vi "AFG3352X.set burst mode.vi"(0 "i ref in":refnum<vi>, 1 "Channel (1: 1)":i32(ring)=1 items=["1"=1, "2"=2], 3 "ms timeout (10000)":i32=10000, 4 "Burst Mode \n(0: Triggered)":i32(ring)=1 items=["Triggered", "Gated"], 5 "error in (no error)":errorcluster) -> (14 "i ref out":refnum<vi>, 17 "timed out":bool, 19 "error out":errorcluster)   [LabVIEW 2014, in "AFG3352X.lvlib"]
doc: "Sets the frequency at my device."
uses:
  AFG3352X.lvlib
  CSlibraries/UtilityLib/UtilityLib.valueStatus.ctl
  CSCore/CSApplicationBaseClasses/AFGBase/AFGBase.directionType.ctl
  CSCore/CSApplicationBaseClasses/DeviceBase/DeviceBase.lvlib
  CSinstr.lib/Agilent 3352X Series/Agilent 3352X Series.lvlib
  CSlibraries/UtilityLib/UtilityLib.lvlib
  CSCore/CSApplicationBaseClasses/AFGBase/AFGBase.lvlib
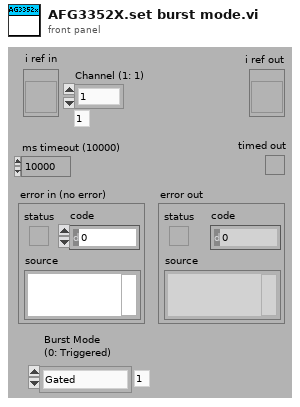
[diagram p1: front panel]
types:
  T1 = typedef "AFGBase.lvlib/AFGBase.directionType.ctl" = enum16{"unknown", "update actual value", "update nominal value", "update both"}
  T2 = typedef "UtilityLib.lvlib/UtilityLib.valueStatus.ctl" = enum16{"no info available", "stand by/off", "on", "warning", "alarm/malfunction", "not implemented", "user action required", "important information", "system default", "control default", "indicator default", "button default"}
  T3 = typedef "AFG3352X.lvlib/AFG3352X.i attribute.ctl" = cluster{"Act2ndValues":cluster{"frequency":dbl, "amplitude":dbl, "phase":dbl, "DCOffset":dbl, "waveformType":T4, "enableOutput":bool, "trigger":i16[], "serviceIDs":cluster{"frequencyID":i32, "amplitudeID":i32, "phaseID":i32, "DCOffsetID":i32, "waveformTypeID":i32, "enableOutputID":i32, "triggerID":i32}, "waveform":cluster{"data":waveform(dbl), "gain":dbl, "offset":dbl, "repetitionRate":dbl, "sampleRate":dbl}}, "Nom2ndValues":cluster{"frequency":dbl, "amplitude":dbl, "phase":dbl, "DCOffset":dbl, "waveformType":T4, "enableOutput":bool, "trigger":i16[], "serviceIDs":cluster{"frequencyID":i32, "amplitudeID":i32, "phaseID":i32, "DCOffsetID":i32, "waveformTypeID":i32, "enableOutputID":i32, "triggerID":i32}, "waveform":cluster{"data":waveform(dbl), "gain":dbl, "offset":dbl, "repetitionRate":dbl, "sampleRate":dbl}}, "DefaultChannel":i32, "ActAddValues":cluster{"Mode1":u16, "serviceIDs":cluster{"Mode1ID":i32, "Mode2ID":i32, "Burst1ID":i32, "Burst2ID":i32}, "Mode2":u16, "Burst1":i32, "Burst2":i32}, "NomAddValues":cluster{"Mode1":u16, "serviceIDs":cluster{"Mode1ID":i32, "Mode2ID":i32, "Burst1ID":i32, "Burst2ID":i32}, "Mode2 2":u16, "Burst1":i32, "Burst2":i32}, "enableBurstMode":bool}
  T4 = typedef "AFGBase.lvlib/AFGBase.waveformType.ctl" = enum16{"sine", "square", "ramp", "pulse", "noise", "DC", "arbitrary", "triangle", "ramp_up", "ramp_down", "amplitude modulation"}
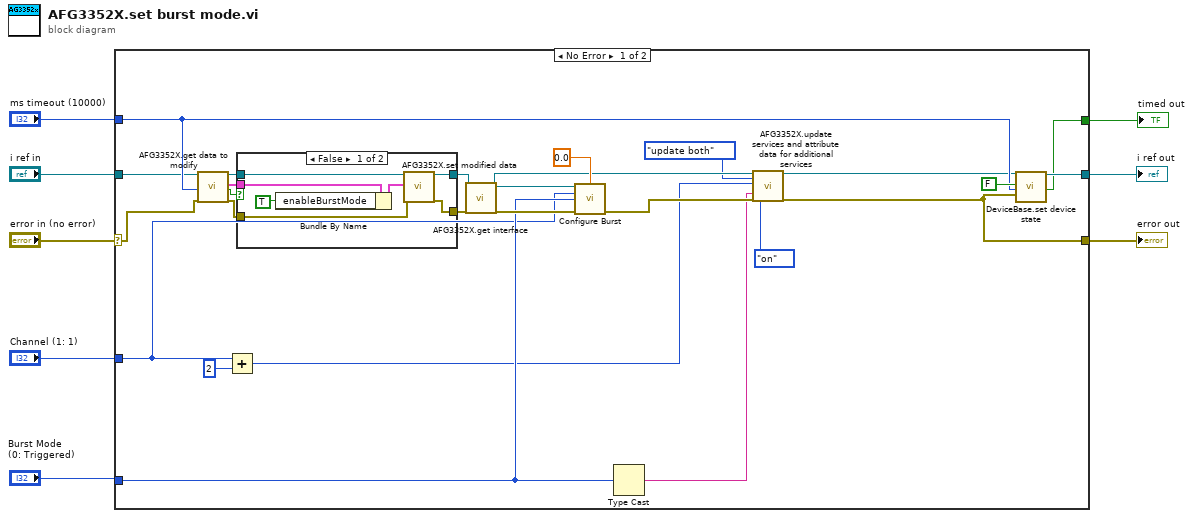
[diagram p0: block diagram]
diagram:
  n1 = case shown="No Error" "error in (no error)" {
    selector: "error in (no error)" -> [w22 w44]
    tunnel: [w34 w45] -> w8
    tunnel: "ms timeout (10000)" -> [w25 _]
    tunnel: "i ref in" -> [w24 w45]
    tunnel: [w16 w44] -> w4
    tunnel: "Burst Mode \n(0: Triggered)" -> [w15 _]
    tunnel: "Channel (1: 1)" -> [w11 _]
    tunnel: [w29 _] -> w1
    frame No Error {
      n2 = call "AFG3352X.get data to modify.vi"("i ref in"=w24, "ms timeout (10000)"=w25, "error in (no error)"=w22) -> ("i ref out"=w27:refnum<vi>, "i attribute"=w28:T3, "timed out"=w20:bool, "error out"=w26:errorcluster)  [unwired: 13 in]
      n3 = Add(x=w11, y=2) -> (x+y=w9:i32)
      n4 = case shown="False" w20 {
        tunnel: w28 -> [w41 _]
        tunnel: w27 -> [w38 w43]
        tunnel: w26 -> [w37 w42]
        tunnel: [w36 w43] -> w23
        tunnel: [w35 w42] -> w21
        frame False {
          n5 = Bundle By Name(cluster=w41, "enableBurstMode"=TRUE) -> (w39:T3)
          n6 = call "AFG3352X.set modified data.vi"("i ref in"=w38, "i attribute"=w39, "error in (no error)"=w37) -> ("i ref out"=w36:refnum<vi>, "error out"=w35:errorcluster)  [unwired: 15 in]
        }
        frame True {
        }
      }
      n7 = call "AFG3352X.get interface.vi"("i ref in"=w23, "error in (no error)"=w21) -> ("i ref out"=w19:refnum<vi>, "interface"=w31:refnum<visa-resource-name>, "error out"=w32:errorcluster)  [unwired: 15 in]
      n8 = call "Configure Burst.vi"("VISA resource name"=w31, "Burst Phase Angle (0 Degree)"=0.0, "Channel (1: 1)"=w11, "Burst Mode (0: Triggered)"=w15, "error in (no error)"=w32) -> ("error out"=w17:errorcluster)  [unwired: 9 in, 1 out]
      n9 = Type Cast(x=w15) -> (*(type *) &x=w14:string)  [unwired: 1 in]
      n10 = call "AFG3352X.update services and attribute data for additional services.vi"("i ref in"=w19, "direction"=AFGBase.directionType."update both", "Service"=w9, "value"=w14, "error in (no error)"=w17, "quality"=UtilityLib.valueStatus."on") -> ("i ref out"=w18:refnum<vi>, "error out"=w16:errorcluster)  [unwired: 11 in, 1 out]
      n11 = call "DeviceBase.set device state.vi"("i ref in"=w18, "implicit"=FALSE, "ms timeout (10000)"=w25, "device error"=w16) -> ("i ref out"=w34:refnum<vi>, "timed out"=w29:bool)  [unwired: 13 in, 1 out]
    }
    frame Error {
    }
  }
  "error out" <- w4
  "i ref out" <- w8
  "timed out" <- w1
